vi "ConfigPath.vi"() -> (3 "ConfigPath":path)   [LabVIEW 2016]
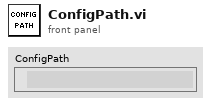
[diagram p1: front panel]
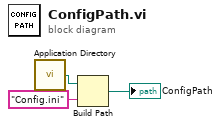
[diagram p0: block diagram]
diagram:
  n1 = call <vilib>:"Application Directory.vi"() -> ("Application Directory"=w1:path)
  n2 = Build Path(base path=w1, name or relative path="Config.ini") -> (appended path=→"ConfigPath":path)
